vi "Error Query.vi"(8 "error in (no error)":errorcluster, 11 "VISA resource name":refnum<visa-resource-name>) -> (0 "error out":errorcluster, 1 "Error Message":string, 2 "Error Code":i32[](array[numeric]), 3 "VISA resource name out":refnum<visa-resource-name>)   [LabVIEW 2023, in "Tektronix AFG 3000 Series.lvlib"]
doc: "Queries the instrument for any errors in the instrument's error queue. It will continue to read errors until all errors have been read from the instrument. Any errors will be returned in the <B>error out</B> control.\n\n<B>Note:</B>\n\nThis VI is called automatically by most driver VIs so it is not usually necessary to call this in an application."
uses:
  Tektronix AFG 3000 Series.lvlib
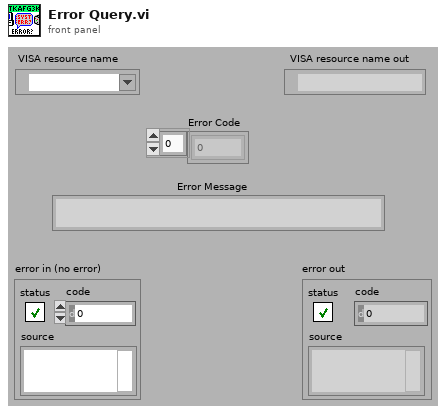
[diagram p1: front panel]
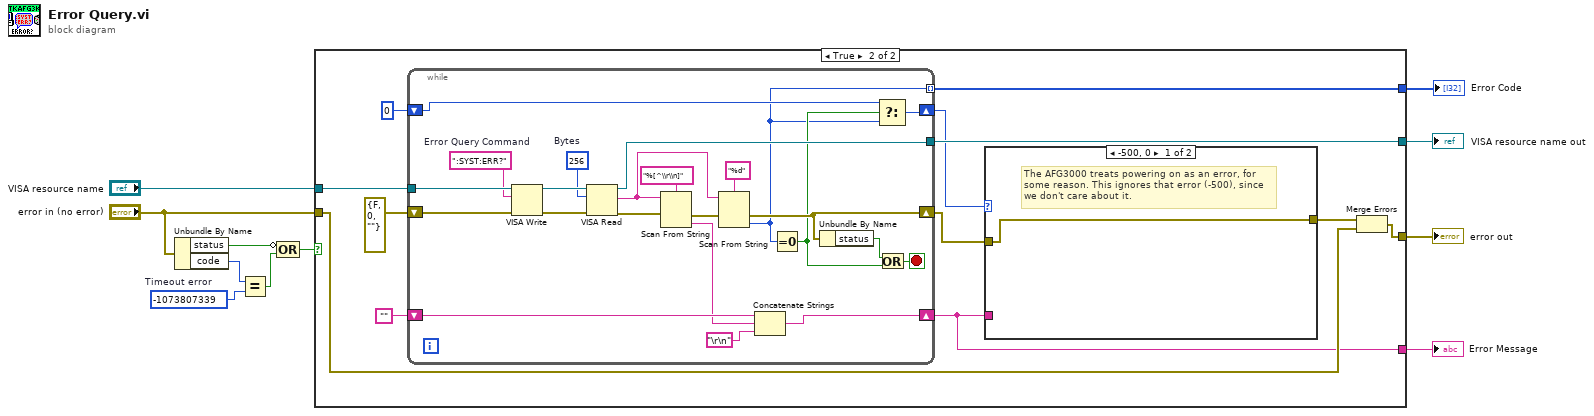
[diagram p0: block diagram]
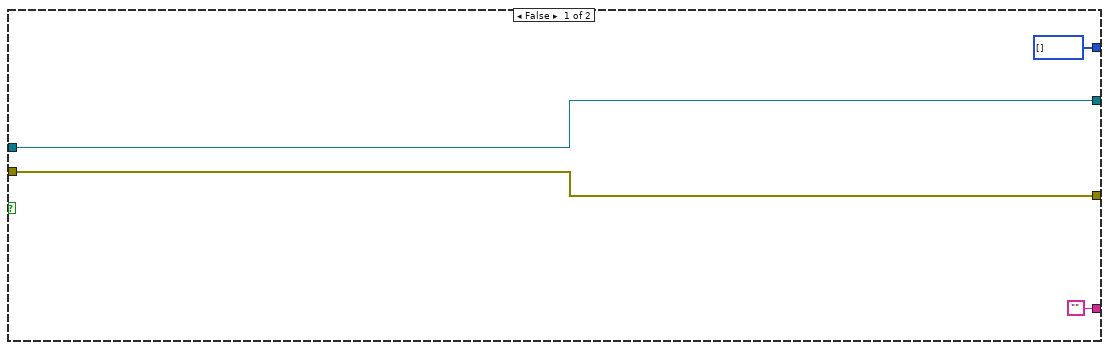
[diagram p2: hidden frame]
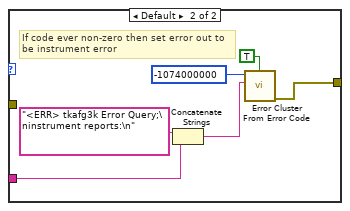
[diagram p3: hidden frame]
diagram:
  w6 = -1073807339  # Timeout error
  n1 = Unbundle By Name("error in (no error)") -> ("status"=w7:bool, "code"=w4:i32)
  n2 = Equal?(x=w4, y=w6) -> (x = y?=w5:bool)
  n3 = Compound Arithmetic op=OR(invert w7, w5) -> (w3:bool)
  n4 = case shown="True" w3 {
    tunnel: [w15 w27] -> w11
    tunnel: "VISA resource name" -> [w15 w26]
    tunnel: "error in (no error)" -> [w14 w21]
    tunnel: [w14 w24] -> w9
    tunnel: ["" w19] -> w2
    tunnel: [i32[] [] w18] -> w1
    frame False {
    }
    frame True {
      n5 = while {
        tunnel: [w57] -> w27
        tunnel: w26 -> [w56]
        shift-right: [w44] -> w19
        shift-left: "" -> [w47]
        shift-right: [w42] -> w16
        shift-left: 0 -> [w43]
        shift-right: [w40] -> w17
        shift-left: errorcluster {"status"=FALSE, "code"=0, "source"=""} ("error in (no error)") -> [w41]
        tunnel: [w35] -> w18 mode=indexing
        stop <- w50 stop-if-true
        w54 = u32 256  # Bytes
        w52 = ":SYST:ERR?"  # Error Query Command
        n6 = VISA Write(VISA resource name=w56, write buffer=w52, error in (no error)=w41) -> (VISA resource name out=w55:refnum<visa-resource-name>, error out=w53:errorcluster)  [unwired: 1 out]
        n7 = VISA Read(VISA resource name=w55, byte count=w54, error in (no error)=w53) -> (VISA resource name out=w57:refnum<visa-resource-name>, read buffer=w48:string, error out=w39:errorcluster)  [unwired: 1 out]
        n8 = Scan From String(format string="%[^\\r\\n]", input string=w48, error in=w39) -> (error out=w38:errorcluster, output 1=w45:string)  [unwired: 1 in, 3 out]
        n9 = Scan From String(format string="%d", input string=w48, error in=w38) -> (error out=w40:errorcluster, output 1=w35:i32)  [unwired: 1 in, 3 out]
        n10 = Concatenate Strings(w47, w45, "\r\n") -> (w44:string)
        n11 = Equal To 0?(x=w35) -> (x = 0?=w36:bool)
        n12 = Unbundle By Name(w40) -> ("status"=w37:bool)
        n13 = Select(t=w43, s=w36, f=w35) -> (s? t:f=w42:i32)
        n14 = Or(x=w37, y=w36) -> (x .or. y?=w50:bool)
      }
      n15 = case shown="-500, 0" w16 {
        tunnel: w19 -> [_ w33]
        tunnel: [w28 w32] -> w22
        tunnel: w17 -> [w28 _]
        frame -500, 0 {
          # "The AFG3000 treats powering on as an error, for some reason. This ignores that error (-500), since we don't care about it."
        }
        frame Default {
          # "If code ever non-zero then set error out to\nbe instrument error"
          n16 = Concatenate Strings("<ERR> tkafg3k Error Query;\ninstrument reports:\n" ("Source"), w33) -> (w29:string)
          n17 = call <vilib>:"Error Cluster From Error Code.vi"("show call chain? (False)"=TRUE ("Status"), "error message (\"\")"=w29, "error code (0)"=-1074000000 ("Code")) -> ("error out"=w32:errorcluster)  [unwired: 1 in, 5 out]
        }
      }
      n18 = Merge Errors(w22, w21) -> (w24:errorcluster)
    }
  }
  "VISA resource name out" <- w11
  "error out" <- w9
  "Error Message" <- w2
  "Error Code" <- w1
